vi "Set and Get Row or Col Head Strings.vi"(6 "Row Or Col":T1=enum."Col", 7 "Mode":T2, 8 "错误输入":errorcluster, 10 "String[]  In":string[](array[string]), 11 "Mlistbox Ref":refnum<vi>) -> (0 "错误输出":errorcluster, 2 "String[] Out":string[](array[string]), 3 "Mlistbox Ref Dup":refnum<vi>)   [LabVIEW 2011, in "Mlistbox Tools.lvlib"]
uses:
  Mlistbox Tools.lvlib
  ListBox/Custom Type/Read and Write Mode.ctl
  Custom Type/Row and Col Option.ctl
  ListBox/Listbox Tool.lvlib
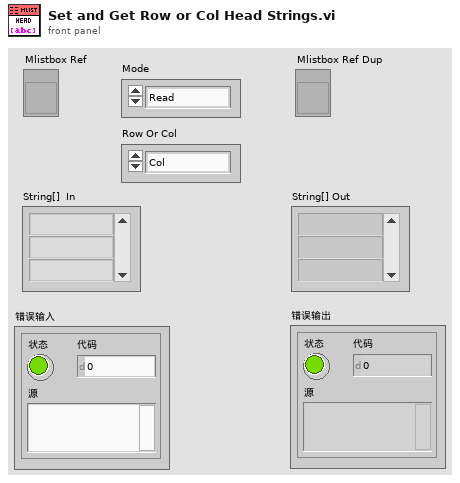
[diagram p1: front panel]
types:
  T1 = typedef "Mlistbox Tools.lvlib/Row and Col Option.ctl" = enum16{"Row", "Col"}
  T2 = typedef "Listbox Tool.lvlib/Read and Write Mode.ctl" = enum16{"Read", "Write"}
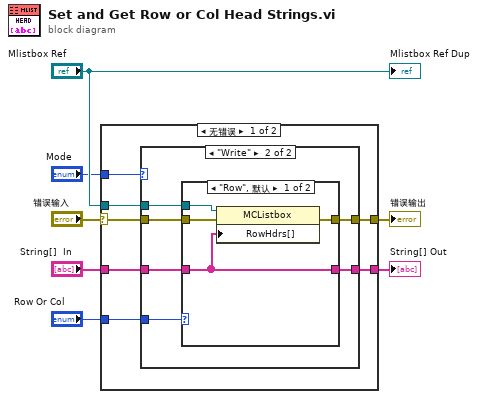
[diagram p0: block diagram]
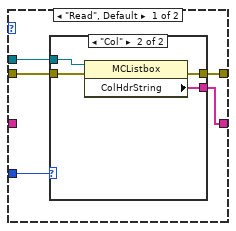
[diagram p2: hidden frame]
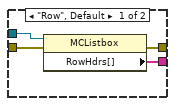
[diagram p3: hidden frame]
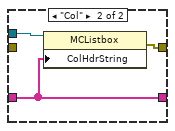
[diagram p4: hidden frame]
diagram:
  n1 = case shown="无错误" "错误输入" {
    selector: "错误输入" -> [w10 w41]
    tunnel: [w9 w41] -> w6
    tunnel: "Mlistbox Ref" -> [w12 _]
    tunnel: "Mode" -> [w14 _]
    tunnel: "Row Or Col" -> [w13 _]
    tunnel: [w11 _] -> w2
    tunnel: "String[]  In" -> [w8 _]
    frame No Error {
      n2 = case shown="\"Write\"" w14 {
        tunnel: w13 -> [w19 w33]
        tunnel: w12 -> [w18 w32]
        tunnel: [w17 w29] -> w11
        tunnel: w10 -> [w16 w28]
        tunnel: [w15 w31] -> w9
        tunnel: w8 -> [_ w30]
        frame "Read", Default {
          n3 = case shown="\"Col\"" w19 {
            tunnel: w18 -> [w20 w27]
            tunnel: [w23 w26] -> w17
            tunnel: w16 -> [w22 w25]
            tunnel: [w21 w24] -> w15
            frame "Row", Default {
              n4 = property class="MCListbox"(reference=w20, error in=w22) -> (error out=w21:errorcluster, "RowHdrs[]"=w23:string[])  [unwired: 1 out]
            }
            frame "Col" {
              n5 = property class="MCListbox"(reference=w27, error in=w25) -> (error out=w24:errorcluster, "ColHdrString"=w26:string[])  [unwired: 1 out]
            }
          }
        }
        frame "Write" {
          n6 = case shown="\"Row\", 默认" w33 {
            tunnel: w32 -> [w35 w40]
            tunnel: [w37 w39] -> w31
            tunnel: w30 -> [w34 w38]
            tunnel: [w34 w38] -> w29
            tunnel: w28 -> [w36 _]
            frame "Row", Default {
              n7 = property class="MCListbox"(reference=w35, error in=w36, "RowHdrs[]"=w34) -> (error out=w37:errorcluster)  [unwired: 1 out]
            }
            frame "Col" {
              n8 = property class="MCListbox"(reference=w40, "ColHdrString"=w38) -> (error out=w39:errorcluster)  [unwired: 1 in, 1 out]
            }
          }
        }
      }
    }
    frame Error {
    }
  }
  "错误输出" <- w6
  "String[] Out" <- w2
  "Mlistbox Ref Dup" <- "Mlistbox Ref"
